vi "send abs move to sample stage.vi"(8 "error in (no error)":errorcluster, 10 "abs position":dbl[unit], 11 "Autofocus in":refnum<class "Autofocus.lvclass">) -> (0 "error out":errorcluster, 3 "Autofocus out":refnum<class "Autofocus.lvclass">)   [LabVIEW 2012, in "Autofocus.lvclass"]
uses:
  Autofocus.lvclass
  <vilib>/Distrio/Murmex/GenericMessage/GenericMessage.lvclass
  Autofocus.lvclass/Autofocus.ctl
  <vilib>/Distrio/Murmex/Message/Message.lvclass
  <vilib>/Distrio/Murmex/Murmex/Murmex.lvclass
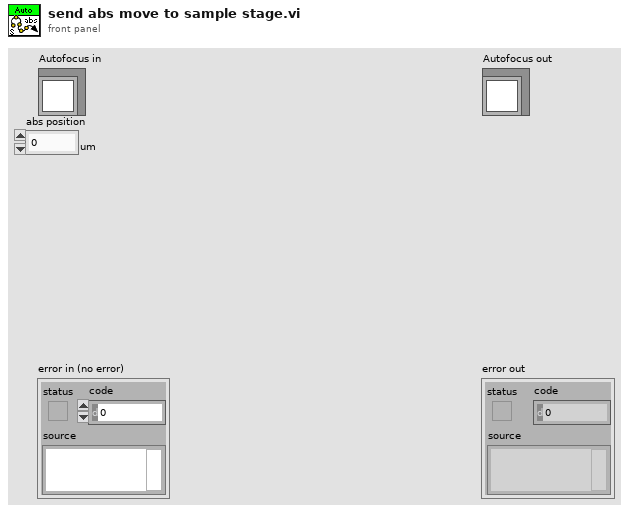
[diagram p1: front panel]
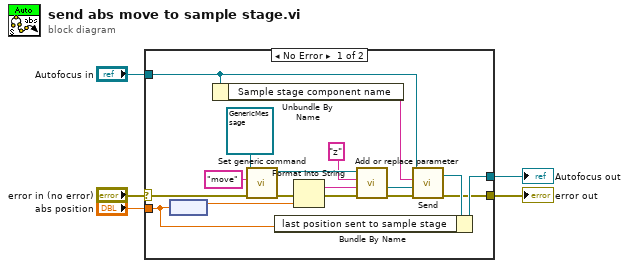
[diagram p0: block diagram]
diagram:
  n1 = case shown="No Error" "error in (no error)" {
    selector: "error in (no error)" -> [w8 w24]
    tunnel: [w7 w24] -> w4
    tunnel: [w9 w23] -> w2
    tunnel: "Autofocus in" -> [w10 w23]
    tunnel: "abs position" -> [w6 _]
    frame No Error {
      n2 = node(w6) -> (w22:dbl)
      n3 = Unbundle By Name(w10) -> ("Sample stage component name"=w19:string)
      n4 = call <vilib>:"Set generic command.vi"("error in (no error)"=w8, "generic command"="move" ("command string"), "GenericMessage in"=refnum<class "GenericMessage.lvclass"> refnum ("Murmex.lvlib:GenericMessage")) -> ("error out"=w18:errorcluster, "GenericMessage out"=w20:refnum<class "GenericMessage.lvclass">)  [unwired: 7 in]
      n5 = Format Into String(error in=w18, w22) -> (resulting string=w14:string, error out=w15:errorcluster)  [unwired: 2 in]
      n6 = call <vilib>:"Add or replace parameter.vi"("error in (no error)"=w15, "value"=w14, "name"="z", "Message in"=w20) -> ("error out"=w12:errorcluster, "Message out"=w11:refnum<class "GenericMessage.lvclass">)  [unwired: 6 in]
      n7 = call <vilib>:"Send.vi"("error in (no error)"=w12, "Message"=w11, "recipient"=w19, "Murmex in"=w10) -> ("error out"=w7:errorcluster, "Murmex out"=w21:refnum<class "Autofocus.lvclass">)  [unwired: 6 in]
      n8 = Bundle By Name(cluster=w21, "last position sent to sample stage"=w6) -> (w9:refnum<class "Autofocus.lvclass">)
    }
    frame Error {
    }
  }
  "error out" <- w4
  "Autofocus out" <- w2
